vi "Get Active Positions.vi"(8 "error in (no error)":errorcluster, 11 "Test Class in":refnum<class "Test Class.lvclass">) -> (0 "error out":errorcluster, 3 "Active Positions":u32[](array[numeric]))   [LabVIEW 2017, in "Test Class.lvclass"]
uses:
  Test Class.lvclass
  Classes/Application/Class/Application.lvclass
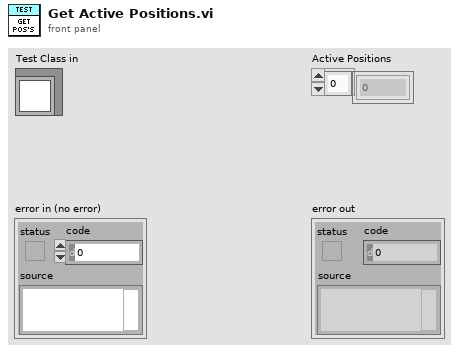
[diagram p1: front panel]
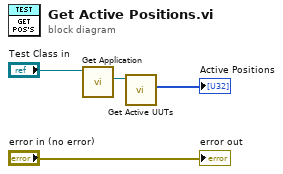
[diagram p0: block diagram]
diagram:
  n1 = call "Get Application.vi"("Test Class in"="Test Class in") -> ("Application.lvlib:Application.lvclass"=w3:refnum<class "Application.lvclass">)  [unwired: 9 in, 1 out]
  n2 = call "Get Active UUTs.vi"("Application in"=w3) -> ("Active Positions"=→"Active Positions":u32[])  [unwired: 8 in, 2 out]
  "error out" <- "error in (no error)"
